vi "PH_Sequencer.PC Action PPPAStateSM.vi"(0 "i ref in":refnum<vi>, 5 "error in (no error)":errorcluster) -> (14 "i ref out":refnum<vi>, 19 "error out":errorcluster)   [LabVIEW 2009, in "PH_Sequencer.lvlib"]
doc: "This is the action of the case PPMAStateSM: depending on the state, it dis- or enbles the set voltage element and writes to GUI and own attributes, if the PUs of the PPMA are running."
uses:
  PH_Sequencer.lvlib
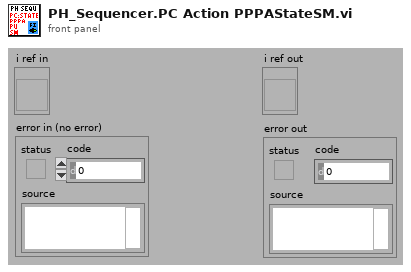
[diagram p1: front panel]
types:
  T1 = typedef "PH_Sequencer.lvlib/PH_Sequencer.i attribute.ctl" = cluster{"GUI Refs":cluster{"Main Off":refnum<vi>, "Fire":refnum<vi>, "Status":refnum<vi>, "Ready":refnum<vi>, "Waiting Time":refnum<vi>, "Timeout":refnum<vi>, "SMs ok":refnum<vi>, "PP DP Ready":refnum<vi>, "Sequencer SM State":refnum<vi>, "PP PA Ready":refnum<vi>, "Calorimeter":refnum<vi>, "Beamline Ready":refnum<vi>, "Clear Beamline":refnum<vi>, "Linkage PPMA Rods":refnum<vi>, "Linkage Current PA":refnum<vi>, "Linkage Current MA":refnum<vi>, "Linkage PPMA Rods 2":refnum<vi>, "Linkage PPMA Rods 3":refnum<vi>, "Linkage Current MA 2":refnum<vi>, "Linkage Current MA 3":refnum<vi>, "PP Booster Ready":refnum<vi>, "PP FR Ready":refnum<vi>, "Timing Ready":refnum<vi>, "State Timing":refnum<vi>, "Force Timing":refnum<vi>, "PSDB Shot Comment":refnum<vi>, "State PA Backreflection":refnum<vi>, "Beamline Z6 Ready":refnum<vi>, "Clear Z6 Beamline":refnum<vi>, "Sequence length":refnum<vi>, "Timing Mode":refnum<vi>, "Slow Trigger Settings":refnum<vi>, "Experiment Description":refnum<vi>, "State PSDB":refnum<vi>, "PSDB Ready":refnum<vi>, "Set PSDB Settings":refnum<vi>, "Get PSDB Info":refnum<vi>, "Take Snapshot":refnum<vi>, "Shottype":refnum<vi>, "Experiment":refnum<vi>, "PA Energy":refnum<vi>, "MA Energy":refnum<vi>, "MA Gain":refnum<vi>}, "Status Info":cluster{"Machine Status":T2, "WaitingTime":i32, "Timeout":bool}, "Readyness":cluster{"Ready to shot":bool, "PP DP Ready":bool, "PPPA Ready":bool, "BL Ready":bool, "PP Booster Ready":bool, "PP FR Ready":bool, "Timing Ready":bool, "BL Z6 Ready":bool, "PSDBReady":bool}, "Instancenames":cluster{"PPMA Rods":string, "PP Current Meas":string, "Beamline":string, "PA Backrefl Meas":string, "Beamline Z6":string}, "Data to read":bool, "Calorimeter":cluster{"Instancename":string, "On":bool, "linked":bool}, "Linkage":cluster{"PPMA Rods":bool, "PP Current Meas":bool, "Beamline":bool, "PA Backrefl Meas":bool, "Beamline Z6":bool}, "PU Info":T3[], "HV Info":T4[], "PSU Info":T5[], "Refs PU on":refnum<vi>[], "Refs Set Voltage PU":refnum<vi>[], "Refs State PU":refnum<vi>[], "Refs State SM PU":refnum<vi>[], "Refs Waiting Time PU":refnum<vi>[], "Refs TO SM PU":refnum<vi>[], "Refs Voltage PU":refnum<vi>[], "Timing":cluster{"Instance":string, "linked":bool, "Status":T2, "Timing Mode":T6, "Slow Trigger Settings":T7, "Info available":cluster{"ext SlowTrigger":bool, "T2":bool, "Mode":bool, "Delay Slow Trigger":bool}}, "GUI Manager Path":string, "Service ID R2S":i32, "PSDB":cluster{"Controller Instance":string, "Controller Status":T2, "Controller linked":bool, "Settings acknowledged":bool, "Current Experiment ID":i16, "Current Shot Type":i16, "Current Comment":string, "Remember Settings":bool, "Write 2 early":bool}, "PSDB Data":cluster{"Main Off?":bool, "Sequence Length":dbl, "Sequence startet":timestamp}, "Beamline":refnum<vi>[], "Powermeter":cluster{"PA":cluster{"Instance":string, "Energy [J]":dbl, "in use":bool}, "MA":cluster{"Instance":string, "Energy [J]":dbl, "in use":bool}, "MA Gain":dbl}}
  T2 = typedef "Status.ctl" = i16
  T3 = typedef "PH_Sequencer.lvlib/PH_Sequencer.PU Info.ctl" = cluster{"Instancename":string, "PU on":bool, "State":T2, "Waiting time":i32, "Set Voltage":dbl, "State SM":string, "Timeout SM":string, "linked":bool}
  T4 = typedef "PH_Sequencer.lvlib/PH_Sequencer.HV Meas Info.ctl" = cluster{"Instancename":string, "linked":bool, "Tagname Meas Voltage":string}
  T5 = typedef "PH_Sequencer.lvlib/PH_Sequencer.PSU Info.ctl" = cluster{"Instancename":string, "linked":bool, "Tagname Applied Voltage":string}
  T6 = typedef "PH_Timing.lvlib/PH_Timing.Timing Mode.ctl" = cluster{"T2 [s]":i16, "Modeselector":enum32{"10 Hz", "0.5 Hz", "Shot"}}
  T7 = typedef "PH_Timing.lvlib/PH_Timing.Slow Trigger Settings.ctl" = cluster{"Delay [ms]":dbl, "externally triggered?":bool}
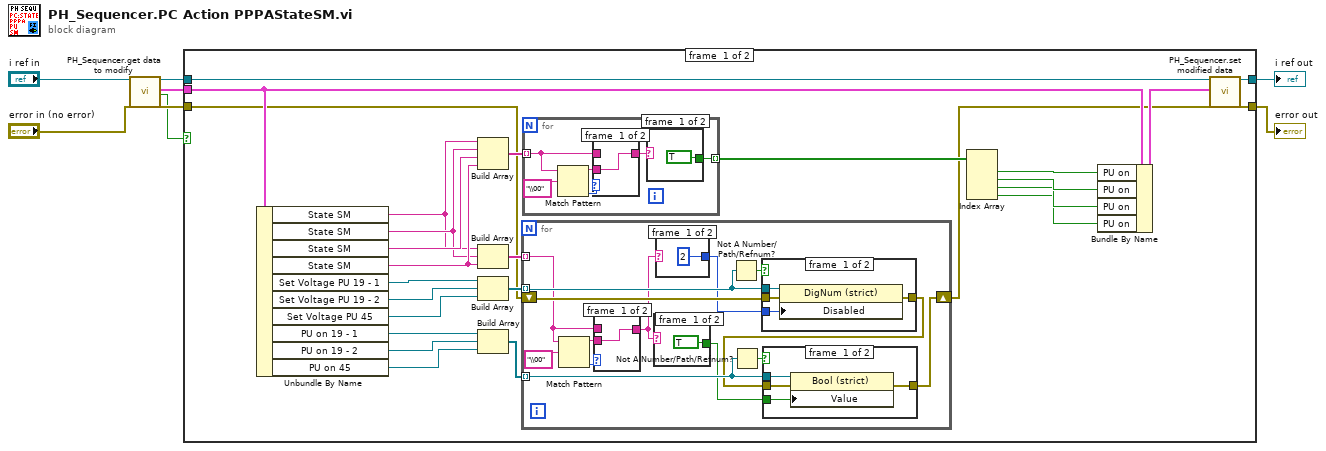
[diagram p0: block diagram]
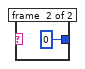
[diagram p3: hidden frame]
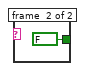
[diagram p5: hidden frame]
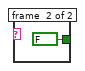
[diagram p8: hidden frame]
diagram:
  n1 = call "PH_Sequencer.get data to modify.vi"("i ref in"="i ref in", "error in (no error)"="error in (no error)") -> ("i ref out"=w4:refnum<vi>, "i attribute"=w2:T1, "timed out"=w1:bool, "error out"=w3:errorcluster)  [unwired: 14 in]
  n2 = case shown="False" w1 {
    tunnel: [w33 w76] -> w8
    tunnel: [w32 w75] -> w6
    tunnel: w4 -> [w31 w76]
    tunnel: w3 -> [w10 w75]
    tunnel: w2 -> [w30 _]
    frame #0 {
      n3 = Unbundle By Name(w30) -> ("State SM"=w11:string, "State SM"=w12:string, "State SM"=w17:string, "State SM"=w16:string, "Set Voltage PU 19 - 1"=w29:refnum<vi>, "Set Voltage PU 19 - 2"=w28:refnum<vi>, "Set Voltage PU 45"=w27:refnum<vi>, "PU on 19 - 1"=w25:refnum<vi>, "PU on 19 - 2"=w24:refnum<vi>, "PU on 45"=w23:refnum<vi>)
      n4 = Build Array(w11, w12, w17, w16) -> (w26:string[])
      n5 = Build Array(w11, w12, w16) -> (w15:string[])
      n6 = Build Array(w29, w28, w27) -> (w14:refnum<vi>[])
      n7 = Build Array(w25, w24, w23) -> (w13:refnum<vi>[])
      n8 = for {
        tunnel: w14 -> [w43] mode=indexing
        shift-right: [w41] -> w9
        shift-left: w10 -> [w48]
        tunnel: w15 -> [w37] mode=indexing
        tunnel: w13 -> [w45] mode=indexing
        n9 = Match Pattern(string=w37, regular expression="\\00" ("search string")) -> (before substring=w38:string, offset past match=w39:i32)  [unwired: 1 in, 2 out]
        n10 = case shown="Default" w39 {
          tunnel: [w49 w50] -> w36
          tunnel: w37 -> [_ w50]
          tunnel: w38 -> [w49 _]
          frame #0 {
          }
          frame #1 {
          }
        }
        n11 = case shown="Default" w36 {
          tunnel: [TRUE FALSE] -> w42
          frame #0 {
          }
          frame #1 {
          }
        }
        n12 = case shown="\"Switch PU on\", \"Wait for Shot Cmd\"" w36 {
          tunnel: [2 0] -> w40
          frame #0 {
          }
          frame #1 {
          }
        }
        n13 = Not A Number/Path/Refnum?(number/path/refnum=w43) -> (NaN/Path/Refnum?=w47:bool)
        n14 = Not A Number/Path/Refnum?(number/path/refnum=w45) -> (NaN/Path/Refnum?=w46:bool)
        n15 = case shown="False" w47 {
          tunnel: w43 -> [w63 _]
          tunnel: w48 -> [w62 w64]
          tunnel: [w61 w64] -> w44
          tunnel: w40 -> [w60 _]
          frame #0 {
            n16 = property class="DigNum (strict)"(reference=w63, error in=w62, "Disabled"=w60) -> (error out=w61:errorcluster)  [unwired: 1 out]
          }
          frame #1 {
          }
        }
        n17 = case shown="False" w46 {
          tunnel: w45 -> [w56 _]
          tunnel: w44 -> [w55 w57]
          tunnel: [w54 w57] -> w41
          tunnel: w42 -> [w53 _]
          frame #0 {
            n18 = property class="Bool (strict)"(reference=w56, error in=w55, "Value"=w53) -> (error out=w54:errorcluster)  [unwired: 1 out]
          }
          frame #1 {
          }
        }
      }
      n19 = for {
        tunnel: w26 -> [w66] mode=indexing
        tunnel: [w70] -> w18 mode=indexing
        n20 = Match Pattern(string=w66, regular expression="\\00" ("search string")) -> (before substring=w68:string, offset past match=w69:i32)  [unwired: 1 in, 2 out]
        n21 = case shown="Default" w69 {
          tunnel: [w71 w72] -> w65
          tunnel: w66 -> [_ w72]
          tunnel: w68 -> [w71 _]
          frame #0 {
          }
          frame #1 {
          }
        }
        n22 = case shown="\"Stand by\", \"no info\"" w65 {
          tunnel: [TRUE FALSE] -> w70
          frame #0 {
          }
          frame #1 {
          }
        }
      }
      n23 = Index Array(array=w18) -> (element #1=w22:bool, element #2=w21:bool, element #3=w20:bool, element #4=w19:bool)  [unwired: 4 in]
      n24 = Bundle By Name(cluster=w30, "PU on"=w22, "PU on"=w21, "PU on"=w20, "PU on"=w19) -> (w34:T1)
      n25 = call "PH_Sequencer.set modified data.vi"("i ref in"=w31, "i attribute"=w34, "error in (no error)"=w9) -> ("i ref out"=w33:refnum<vi>, "error out"=w32:errorcluster)  [unwired: 15 in]
    }
    frame #1 {
    }
  }
  "i ref out" <- w8
  "error out" <- w6
